vi "ZC_gysh.vi"(0 "name":string, 1 "LabVIEW Web Service Request":refnum<class "Web Request.lvclass"> caption="LabVIEW Web服务请求", 2 "id":string, 3 "chuanzhen":string, 4 "number":string, 5 "zizhi":string, 7 "dizhi":string, 9 "action":string, 10 "key":string, 11 "dianhua":string, 12 "wangzhi":string, 13 "Email":string, 14 "beizhu":string) -> (6 "error":errorcluster)   [LabVIEW 2017]
uses:
  <vilib>/wsapi/Web Request.lvclass
panel:
  out "postdata":string caption="post数据"
  out "error out":errorcluster caption="错误输出"
  # "Web服务请求输入接线端用于调用“Web服务”选板的VI。除非不需要访问该选板，否则不要在连线板上删除这个输入接线端。"
  # "添加至连线板的每一个其他输入控件，在URL中对应于一个输入。如需在接线端模式输出（默认设置）下包含显示控件，则该显示控件必须与连线板相连。"
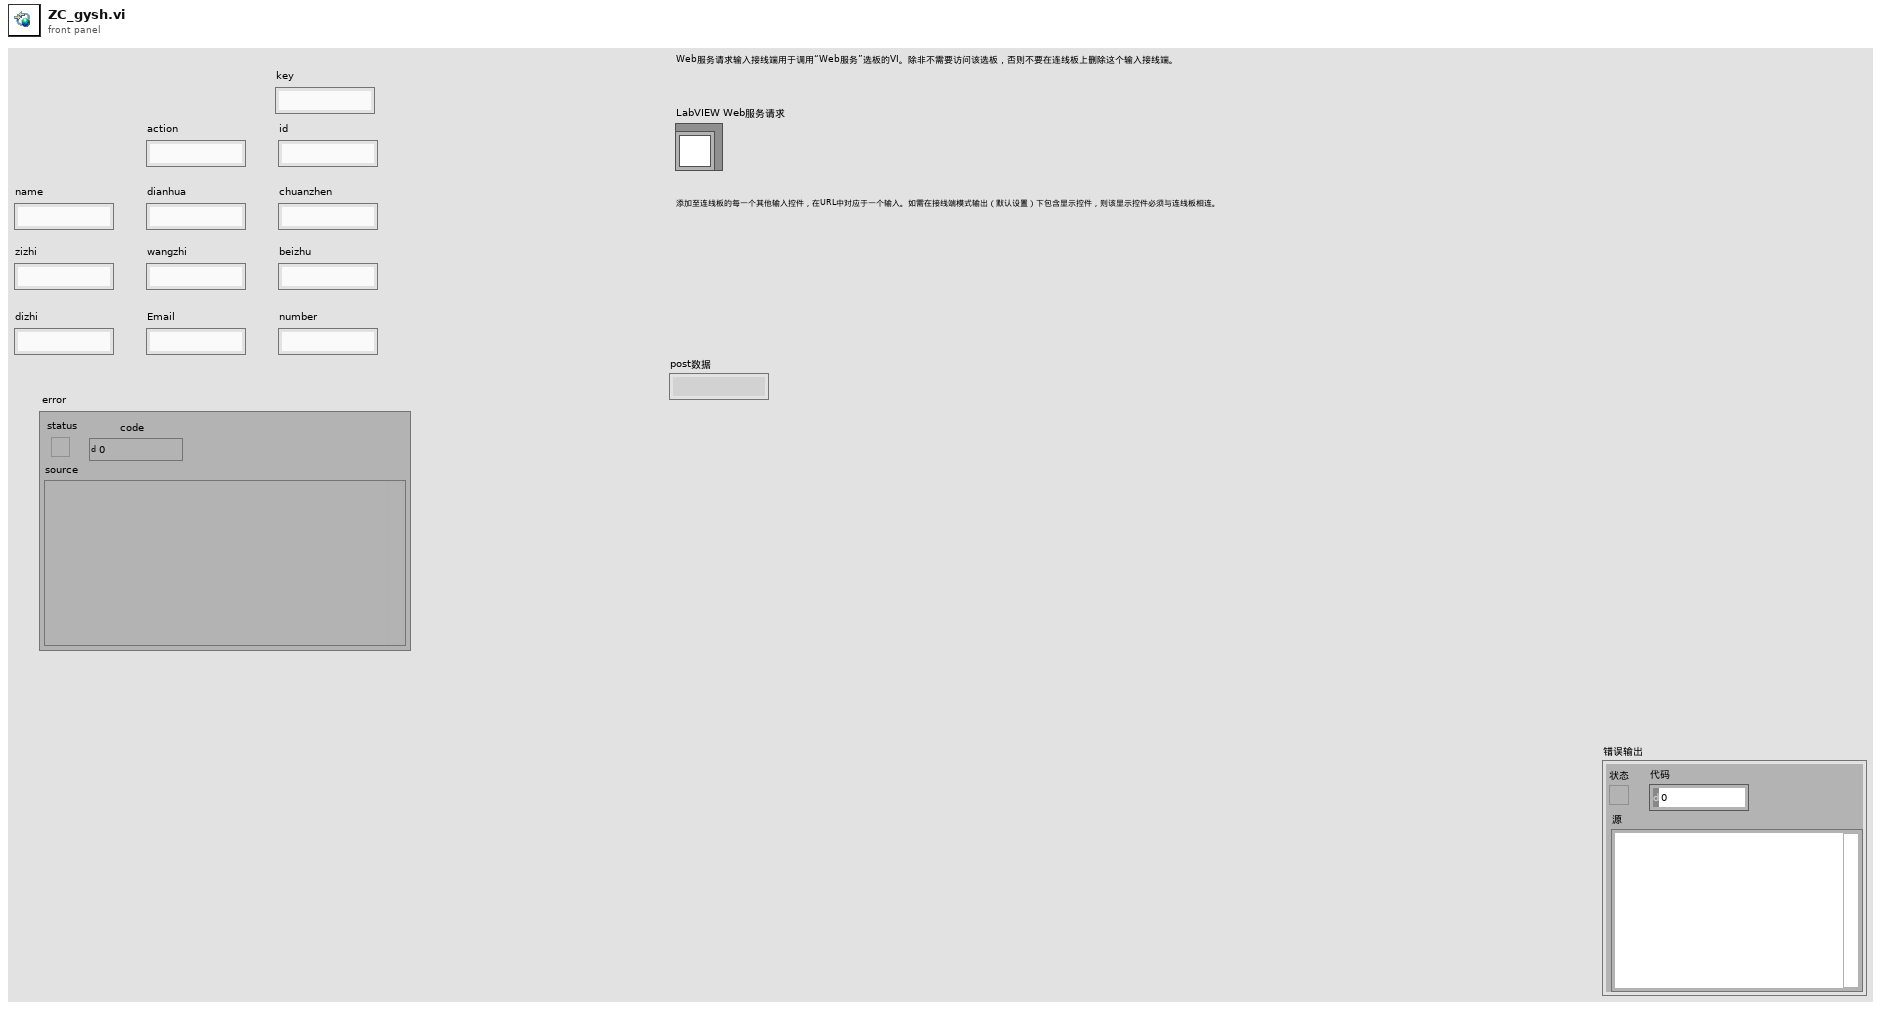
[diagram p1: front panel]
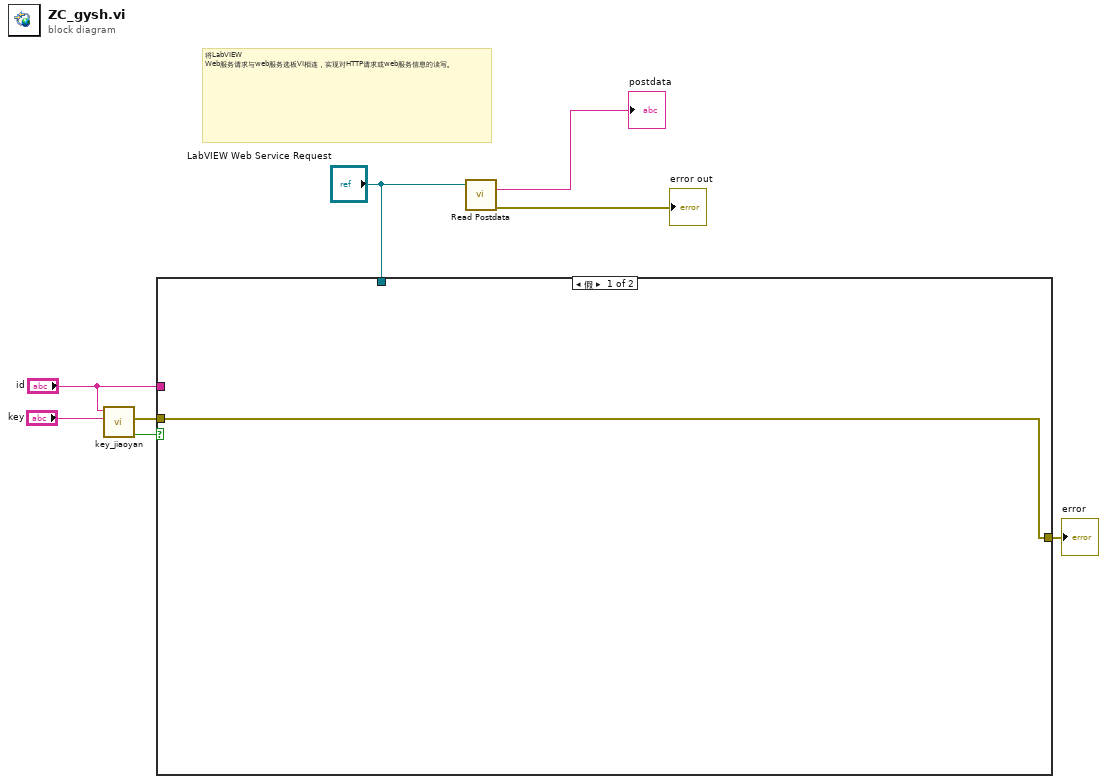
[diagram p0: block diagram]
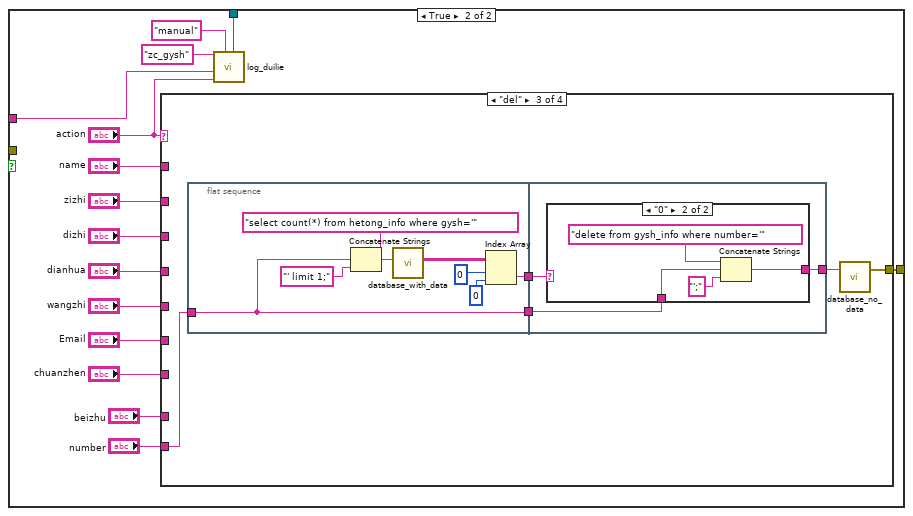
[diagram p2: hidden frame]
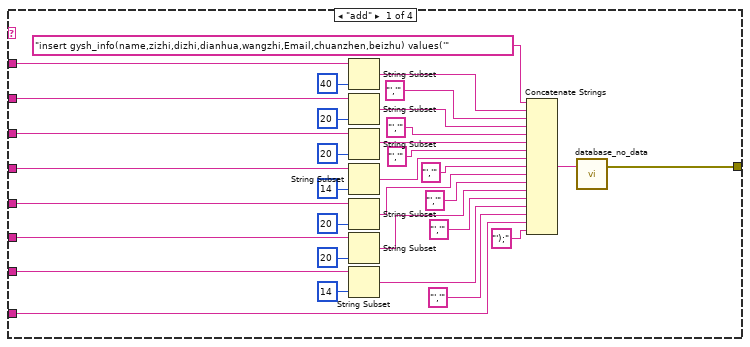
[diagram p3: hidden frame]
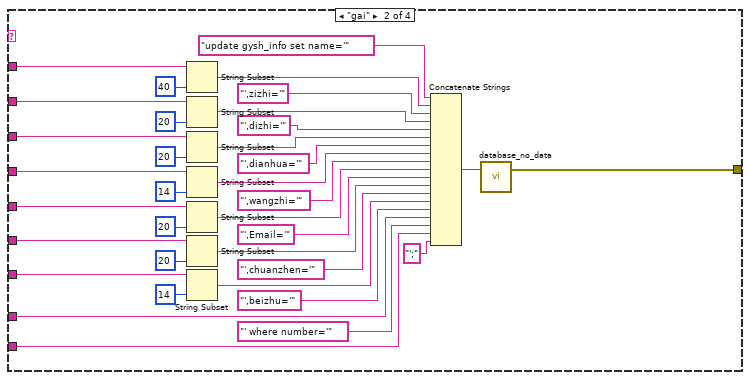
[diagram p4: hidden frame]
diagram:
  # "将LabVIEW Web服务请求与web服务选板VI相连，实现对HTTP请求或web服务信息的读写。"
  n1 = call "key_jiaoyan.vi"("key_client"="key", "gonghao"="id") -> ("jy"=w2:bool, "error"=w1:errorcluster)  [unwired: 8 in]
  n2 = case shown="假" w2 {
    tunnel: [w9 w24] -> w7
    tunnel: "LabVIEW Web Service Request" -> [_ w12]
    tunnel: "id" -> [_ w10]
    tunnel: w1 -> [w9 _]
    frame False {
    }
    frame True {
      n3 = case shown="\"del\"" "action" {
        tunnel: [w33 w78 w93 _] -> w24
        tunnel: "chuanzhen" -> [w32 w77 _ _]
        tunnel: "beizhu" -> [w31 w76 _ _]
        tunnel: "Email" -> [w30 w75 _ _]
        tunnel: "wangzhi" -> [w29 w74 _ _]
        tunnel: "dianhua" -> [w28 w73 _ _]
        tunnel: "dizhi" -> [w27 w72 _ _]
        tunnel: "zizhi" -> [w26 w71 _ _]
        tunnel: "name" -> [w25 w70 _ _]
        tunnel: "number" -> [_ w64 w94 _]
        frame "add" {
          n4 = String Subset(string=w25, length (rest)=40 ("长度（剩余）")) -> (substring=w53:string)  [unwired: 1 in]
          n5 = String Subset(string=w26, length (rest)=20 ("长度（剩余）")) -> (substring=w51:string)  [unwired: 1 in]
          n6 = String Subset(string=w27, length (rest)=20 ("长度（剩余）")) -> (substring=w49:string)  [unwired: 1 in]
          n7 = String Subset(string=w28, length (rest)=14 ("长度（剩余）")) -> (substring=w47:string)  [unwired: 1 in]
          n8 = String Subset(string=w29, length (rest)=20 ("长度（剩余）")) -> (substring=w42:string)  [unwired: 1 in]
          n9 = String Subset(string=w30, length (rest)=20 ("长度（剩余）")) -> (substring=w39:string)  [unwired: 1 in]
          n10 = String Subset(string=w32, length (rest)=14 ("长度（剩余）")) -> (substring=w36:string)  [unwired: 1 in]
          n11 = Concatenate Strings("insert gysh_info(name,zizhi,dizhi,dianhua,wangzhi,Email,chuanzhen,beizhu) values('" ("格式字符串"), w53, "','" ("字符串"), w51, "','" ("字符串"), w49, "','" ("字符串"), w47, "','" ("字符串"), w42, "','" ("字符串"), w39, "','" ("字符串"), w36, "','" ("字符串"), w31, "');" ("字符串")) -> (w34:string)
          n12 = call "database_no_data.vi"("input"=w34) -> ("error"=w33:errorcluster)  [unwired: 2 in]
        }
        frame "gai" {
          n13 = String Subset(string=w70, length (rest)=40 ("长度（剩余）")) -> (substring=w91:string)  [unwired: 1 in]
          n14 = String Subset(string=w71, length (rest)=20 ("长度（剩余）")) -> (substring=w89:string)  [unwired: 1 in]
          n15 = String Subset(string=w72, length (rest)=20 ("长度（剩余）")) -> (substring=w68:string)  [unwired: 1 in]
          n16 = String Subset(string=w73, length (rest)=14 ("长度（剩余）")) -> (substring=w86:string)  [unwired: 1 in]
          n17 = String Subset(string=w74, length (rest)=20 ("长度（剩余）")) -> (substring=w84:string)  [unwired: 1 in]
          n18 = String Subset(string=w75, length (rest)=20 ("长度（剩余）")) -> (substring=w82:string)  [unwired: 1 in]
          n19 = String Subset(string=w77, length (rest)=14 ("长度（剩余）")) -> (substring=w81:string)  [unwired: 1 in]
          n20 = Concatenate Strings("update gysh_info set name='" ("格式字符串"), w91, "',zizhi='" ("字符串"), w89, "',dizhi='" ("字符串"), w68, "',dianhua='" ("字符串"), w86, "',wangzhi='" ("字符串"), w84, "',Email='" ("字符串"), w82, "',chuanzhen='" ("字符串"), w81, "',beizhu='" ("字符串"), w76, "' where number='" ("字符串"), w64, "';" ("字符串")) -> (w79:string)
          n21 = call "database_no_data.vi"("input"=w79) -> ("error"=w78:errorcluster)  [unwired: 2 in]
        }
        frame "del" {
          n22 = flat-sequence {
            tunnel: w94 -> [w103]
            tunnel: [w103] -> w97
            tunnel: [w98] -> w96
            tunnel: [w108] -> w95
            tunnel: w97 -> [w107]
            tunnel: w96 -> [w106]
            frame #0 {
              n23 = Concatenate Strings("select count(*) from hetong_info where gysh='" ("格式字符串"), w103, "' limit 1;" ("字符串")) -> (w102:string)
              n24 = call "database_with_data.vi"("input"=w102) -> ("Data"=w99:string[][])  [unwired: 9 in, 1 out]
              n25 = Index Array(array=w99, index (row)=0 ("索引 (行)"), index (col)=0 ("禁用的索引 (列)")) -> (element=w98:string)
            }
            frame #1 {
              n26 = case shown="\"0\"" w106 {
                tunnel: [_ w110] -> w108
                tunnel: w107 -> [_ w109]
                frame "假", Default {
                }
                frame "0" {
                  n27 = Concatenate Strings("delete from gysh_info where number='" ("格式字符串"), w109, "';" ("字符串")) -> (w110:string)
                }
              }
            }
          }
          n28 = call "database_no_data.vi"("input"=w95) -> ("error"=w93:errorcluster)  [unwired: 2 in]
        }
        frame Default {
        }
      }
      n29 = call "log_duilie.vi"("LabVIEW Web Service Request"=w12, "type"="manual", "action"="action", "user"=w10, "yw"="zc_gysh") -> ()  [unwired: 7 in]
    }
  }
  "error" <- w7
  n30 = call <vilib>:"Read Postdata.vi"("LabVIEW Web Service Request"="LabVIEW Web Service Request") -> ("postdata"=→"postdata":string, "error out"=→"error out":errorcluster)  [unwired: 12 in, 1 out]
